vi "Convert CD Reference to Pointer.vi"(8 "error in (no error)":errorcluster, 11 "Item Ref in":T1 format="%.0x") -> (0 "error out":errorcluster, 2 ".NET Refnum out":refnum<k24>, 3 "Item Ref out":T1 format="%.0x")   [LabVIEW 2018, in "FPGA Addon Shared.lvlib"]
uses:
  FPGA Addon Shared.lvlib
  <vilib>/NI Veristand/Custom Device API/Custom Device Item Ref.ctl
  NationalInstruments.VeriStand.SystemStorage
  NationalInstruments.VeriStand.SystemDefinitionAPI
  <vilib>/NI Veristand/Custom Device API/Custom Device API.lvlib
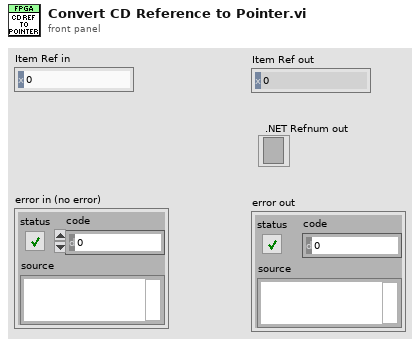
[diagram p1: front panel]
types:
  T1 = typedef "Custom Device API.lvlib/Custom Device Item Ref.ctl" = u64
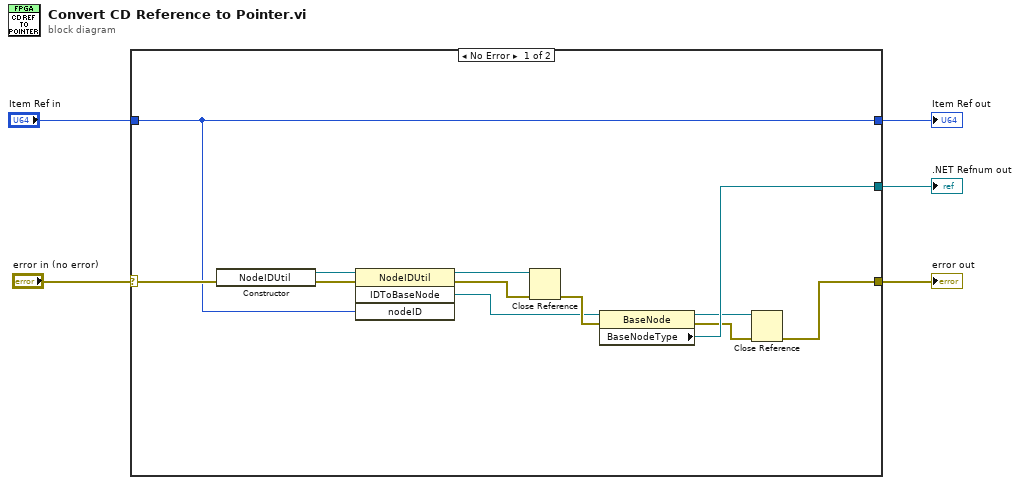
[diagram p0: block diagram]
diagram:
  n1 = case shown="No Error" "error in (no error)" {
    selector: "error in (no error)" -> [w8 w19]
    tunnel: "Item Ref in" -> [w6 w18]
    tunnel: [w17 _] -> w4
    tunnel: [w7 w19] -> w1
    tunnel: [w6 w18] -> w2
    frame No Error {
      n2 = constructor class="NodeIDUtil"(error in=w8) -> (reference out=w9:refnum<k24>, error out=w10:errorcluster)  [unwired: 2 in, 1 out]
      n3 = invoke class="NodeIDUtil" method="IDToBaseNode"(reference=w9, error in=w10, "nodeID"=w6) -> (reference out=w14:refnum<k24>, error out=w12:errorcluster, "IDToBaseNode"=w11:refnum<k24>)  [unwired: 1 in, 1 out]
      n4 = Close Reference(reference=w14, error in (no error)=w12) -> (error out=w13:errorcluster)
      n5 = property class="BaseNode"(reference=w11, error in=w13) -> (reference out=w15:refnum<k24>, error out=w16:errorcluster, "BaseNodeType"=w17:refnum<k24>)
      n6 = Close Reference(reference=w15, error in (no error)=w16) -> (error out=w7:errorcluster)
    }
    frame Error {
    }
  }
  ".NET Refnum out" <- w4
  "Item Ref out" <- w2
  "error out" <- w1
